vi "leapmotion.vi"() -> ()   [LabVIEW 2016]
uses:
  Controls/recognize hands data.ctl
  <vilib>/registry/registry.llb/Registry RtKey.ctl
  <vilib>/registry/registry.llb/Read Registry Value Simple STR.vi
panel:
  out "数字":i32[](array[numeric])
  out "Reconze  hands":T1
  out "fingerdata":T2
  in  "停止":bool
  out "String/Binary data":string="TYPE_THUMB0\nTYPE_INDEX72\nTYPE_MIDDLE67\nTYPE_RING57\nTYPE_PINKY59\n" caption="字符串/二进制数据"
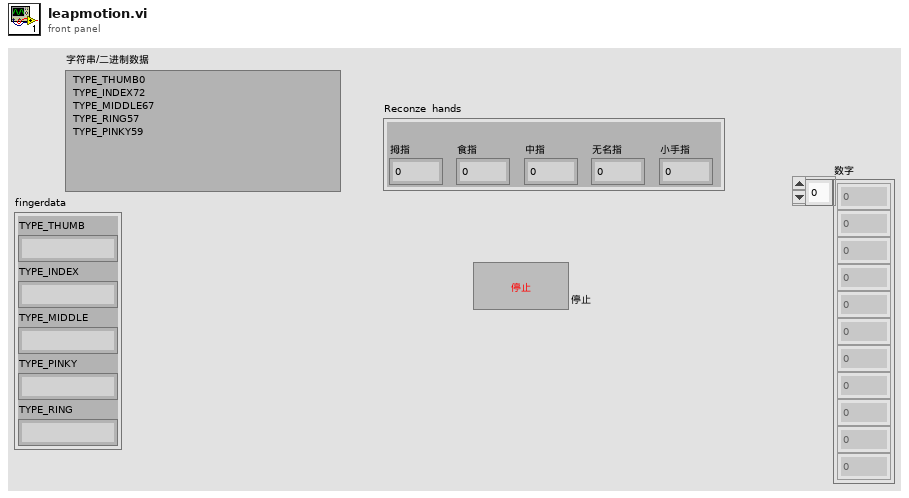
[diagram p1: front panel]
types:
  T1 = typedef "recognize hands data.ctl" = cluster{"小手指":sgl, "无名指":sgl, "中指":sgl, "食指":sgl, "拇指":sgl}
  T2 = cluster{"TYPE_THUMB":string, "TYPE_INDEX":string, "TYPE_MIDDLE":string, "TYPE_PINKY":string, "TYPE_RING":string}
  T3 = typedef "Registry RtKey.ctl" = enum32{"HKEY_CLASSES_ROOT", "HKEY_CURRENT_USER", "HKEY_LOCAL_MACHINE", "HKEY_USERS", "HKEY_PERFORMANCE_DATA", "HKEY_CURRENT_CONFIG", "HKEY_DYN_DATA"}
  T4 = typedef "Registry refnum.ctl" = refnum<k1>
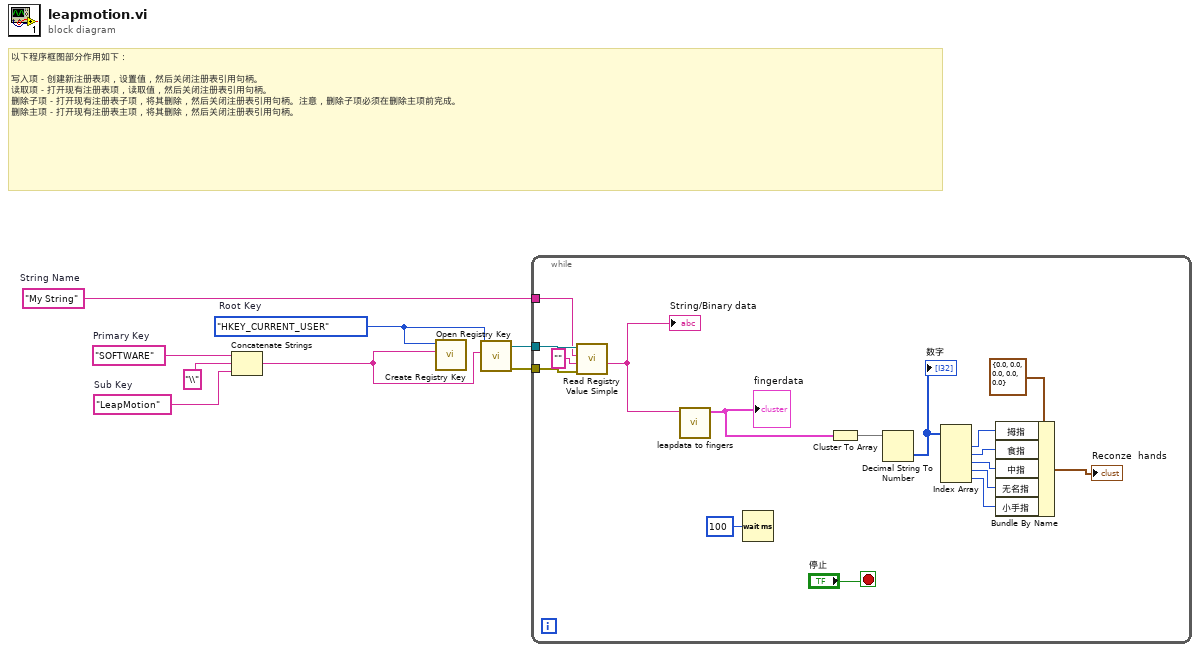
[diagram p0: block diagram]
diagram:
  w6 = "LeapMotion"  # Sub Key
  w4 = "SOFTWARE"  # Primary Key
  w5 = "My String"  # String Name
  w1 = Registry_RtKey."HKEY_CURRENT_USER"  # Root Key
  # "以下程序框图部分作用如下：\n\n写入项－创建新注册表项，设置值，然后关闭注册表引用句柄。\n读取项－打开现有注册表项，读取值，然后关闭注册表引用句柄。\n删除子项－打开现有注册表子项，将其删除，然后关闭注册表引用句柄。注意，删除子项必须在删除主项前完成。\n删除主项－打开现有注册表主项，将其删除，然后关闭注册表引用句柄。"
  n1 = Concatenate Strings(w4, "\\", w6) -> (w2:string)
  n2 = call <vilib>:"Create Registry Key.vi"("subkey"=w2, "root key (HKEY_LOCAL_MACHINE)"=w1) -> ()  [unwired: 7 in, 3 out]
  n3 = call <vilib>:"Open Registry Key.vi"("subkey"=w2, "root key (HKEY_LOCAL_MACHINE)"=w1) -> ("error out"=w7:errorcluster, "refnum out"=w8:T4)  [unwired: 8 in]
  n4 = while {
    tunnel: w8 -> [w25]
    tunnel: w7 -> [w24]
    tunnel: w5 -> [w23]
    stop <- "停止" stop-if-true
    n5 = call-poly <vilib>:"Read Registry Value Simple.vi"("error in (no error)"=w24, "default data"="", "value"=w23, "refnum"=w25) -> ("String/Binary data"=w20:string)  [unwired: 2 in, 3 out]
    "String/Binary data" <- w20
    n6 = call "leapdata to fingers.vi"("leapdata in"=w20) -> ("fingerdata"=w19:T2)  [unwired: 9 in, 1 out]
    "fingerdata" <- w19
    n7 = Wait (ms)(milliseconds to wait=u32 100 ("等待时间（毫秒）")) -> ()  [unwired: 1 out]
    n8 = Cluster To Array(cluster=w19) -> (array=w17:string[])
    n9 = Decimal String To Number(string=w17) -> (number=w15:i32[])  [unwired: 2 in, 1 out]
    "数字" <- w15
    n10 = Index Array(array=w15) -> (element #1=w14:i32, element #2=w13:i32, element #3=w12:i32, element #4=w11:i32, element #5=w10:i32)  [unwired: 5 in]
    n11 = Bundle By Name(cluster=T1 {"小手指"=0.0, "无名指"=0.0, "中指"=0.0, "食指"=0.0, "拇指"=0.0} ("Reconze  hands"), "拇指"=w14, "食指"=w13, "中指"=w12, "无名指"=w11, "小手指"=w10) -> (→"Reconze  hands":T1)
  }
